vi "acqEngineHistoryStorage (U128).vi"(4 "ready for output":bool=TRUE, 7 "FIFO Out":refnum<k21>, 8 "PostTrigComplete":bool, 9 "AcqInProgress":bool, 10 "states":T1, 11 "Input Data":i16[](array[numeric])=[0, 0, 0, 0, 0, 0, 0, 0]) -> (0 "flushed":bool, 1 "valid":bool, 3 "Output Data":i16[](array[numeric]))   [LabVIEW 2011]
uses:
  <instrlib>/FlexRIO/Libraries/Acquisition Engine/FPGA/Interface/acqEngineStates v1.ctl
  <vilib>/rvi/DataTransferAndStorage/Container/Common/niFpgaContainerExecOnDevCompGetState.vi
  <vilib>/rvi/FIFO/Fifo_Resource/nirvififoEmulationSetSize.vi
  <vilib>/rvi/DataTransferAndStorage/Container/Common/niFpgaContainerGetUniqueNameForEmu.vi
  <vilib>/rvi/interface/RandomDataEmulation/nirviRandomDataFPGAFIFO.vi
  <vilib>/rvi/interface/RandomDataEmulation/niFpgaRandomDataHandleErrors.vi
  <vilib>/rvi/eio/common/nirviEmuReportErrorAndStop.vi
  <vilib>/rvi/FXPMathLib/basic elements/FxpDiscreteDelay/XNode/nifxpmath_DiscreteDelay.xnode
  <vilib>/rvi/DataTransferAndStorage/Container/XNode/niFpgaContainer.xnode
  <vilib>/rvi/FIFO/Fifo_Resource/niFpgaFifoEmulationRefIn.vi
  <instrlib>/FlexRIO/Libraries/Flexible Record Storage/Flexible Record Storage.lvlib
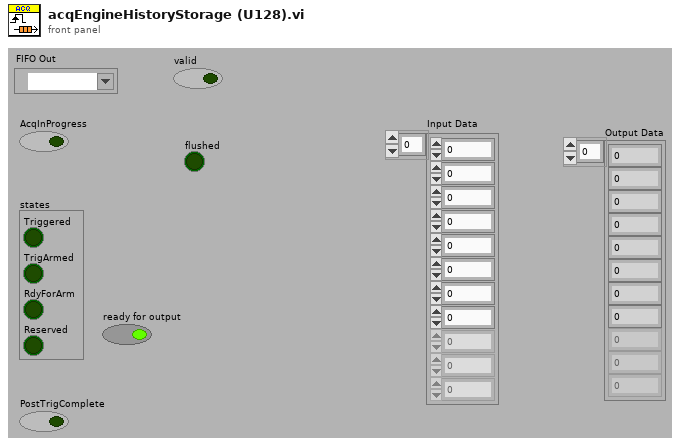
[diagram p1: front panel]
types:
  T1 = typedef "acqEngineStates v1.ctl" = cluster{"Triggered":bool, "TrigArmed":bool, "RdyForArm":bool, "Reserved":bool}
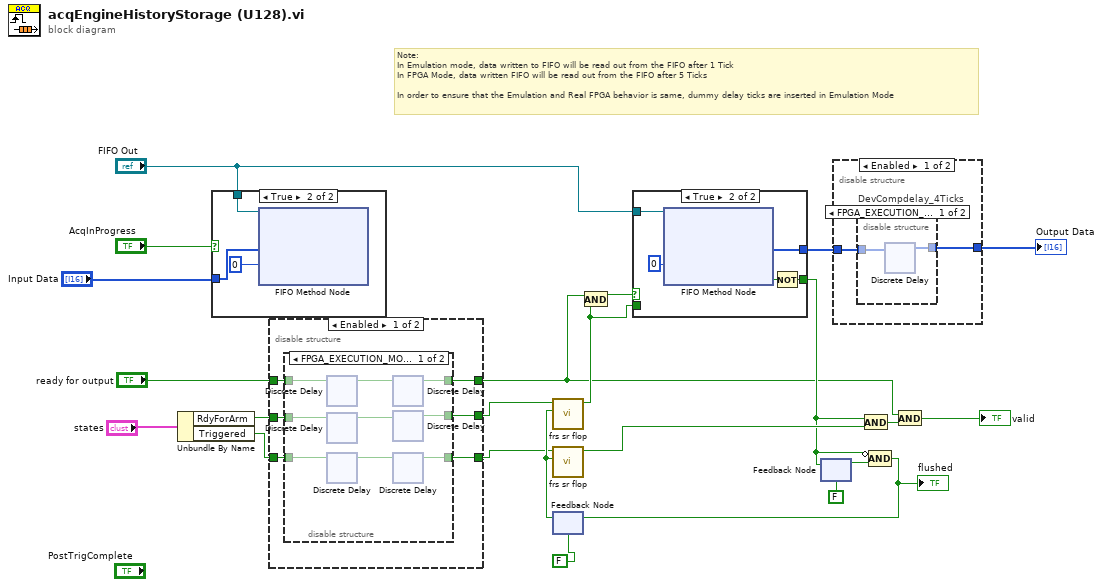
[diagram p0: block diagram]
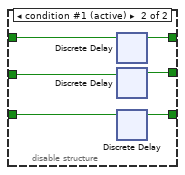
[diagram p2: hidden frame]
diagram:
  # "Note:\nIn Emulation mode, data written to FIFO will be read out from the FIFO after 1 Tick\nIn FPGA Mode, data written FIFO will be read out from the FIFO after 5 Ticks\n\nIn order to ensure that the Emulation and Real FPGA behavior is same, dummy delay ticks are inserted in Emulation Mode"
  n1 = Unbundle By Name("states") -> ("RdyForArm"=w19:bool, "Triggered"=w17:bool)
  n2 = case shown="True" "AcqInProgress" {
    tunnel: "FIFO Out" -> [_ w26]
    tunnel: "Input Data" -> [_ w25]
    frame False {
    }
    frame True {
      n3 = xnode ("FIFO Method Node")("Element"=w25, "Timeout"=0, "FIFO In"=w26) -> ()  [unwired: 2 out]
    }
  }
  n4 = disable-structure shown="Enabled" {
    disable-tunnel: w19 -> [w32 w49]
    disable-tunnel: w17 -> [w31 w48]
    disable-tunnel: "ready for output" -> [w30 w50]
    disable-tunnel: [w29 w49] -> w5
    disable-tunnel: [w28 w50] -> w4
    disable-tunnel: [w27 w48] -> w3
    frame Enabled {
      n5 = disable-structure shown="FPGA_EXECUTION_MODE==DEV_COMPUTER_SIM_IO, default" {
        disable-tunnel: w32 -> [w41 w47]
        disable-tunnel: w31 -> [w40 w46]
        disable-tunnel: w30 -> [w39 w45]
        disable-tunnel: [w38 w44] -> w29
        disable-tunnel: [w37 w43] -> w28
        disable-tunnel: [w36 w42] -> w27
        frame condition #0 {
          n6 = xnode "Discrete Delay"("D"=w39) -> ("Q"=w35:bool)
          n7 = xnode "Discrete Delay"("D"=w41) -> ("Q"=w34:bool)
          n8 = xnode "Discrete Delay"("D"=w40) -> ("Q"=w33:bool)
          n9 = xnode "Discrete Delay"("D"=w35) -> ("Q"=w37:bool)
          n10 = xnode "Discrete Delay"("D"=w34) -> ("Q"=w38:bool)
          n11 = xnode "Discrete Delay"("D"=w33) -> ("Q"=w36:bool)
        }
        frame condition #1 (active) {
          n12 = xnode "Discrete Delay"("D"=w45) -> ("Q"=w43:bool)
          n13 = xnode "Discrete Delay"("D"=w47) -> ("Q"=w44:bool)
          n14 = xnode "Discrete Delay"("D"=w46) -> ("Q"=w42:bool)
        }
      }
    }
    frame Disabled {
    }
  }
  n15 = feedback #1(FALSE) -> (w11:bool)
  n16 = call <instrlib>:"frs sr flop.vi"("r"=w11, "s"=w5) -> ("out"=w9:bool)  [unwired: 7 in]
  n17 = call <instrlib>:"frs sr flop.vi"("r"=w11, "s"=w3) -> ("out"=w16:bool)  [unwired: 7 in]
  n18 = And(x=w4, y=w9) -> (x .and. y?=w10:bool)
  n19 = case shown="True" w10 {
    tunnel: "FIFO Out" -> [_ w56]
    tunnel: [_ w55] -> w2
    tunnel: [w51 w54] -> w13
    tunnel: w9 -> [w51 _]
    frame False {
    }
    frame True {
      n20 = xnode ("FIFO Method Node")("Timeout"=0, "FIFO In"=w56) -> ("Element"=w55:i16[], "Timed Out?"=w53:bool)  [unwired: 1 out]
      n21 = Not(x=w53) -> (.not. x?=w54:bool)
    }
  }
  n22 = feedback #2(FALSE) -> (w15:bool)
  n23 = feedback-in #2(w13) -> ()
  n24 = disable-structure shown="Enabled" {
    disable-tunnel: w2 -> [w58 w62]
    disable-tunnel: [w57 w62] -> w1
    frame Enabled {
      n25 = disable-structure "DevCompdelay_4Ticks" shown="FPGA_EXECUTION_MODE==DEV_COMPUTER_SIM_IO, default" {
        disable-tunnel: w58 -> [w60 w61]
        disable-tunnel: [w59 w61] -> w57
        frame condition #0 {
          n26 = xnode "Discrete Delay"("D"=w60) -> ("Q"=w59:i16[])
        }
        frame condition #1 (active) {
        }
      }
    }
    frame Disabled {
    }
  }
  "Output Data" <- w1
  n27 = And(x=w13, y=w16) -> (x .and. y?=w18:bool)
  n28 = Compound Arithmetic op=AND(invert w13, w15) -> (w12:bool)
  "flushed" <- w12
  n29 = feedback-in #1(w12) -> ()
  n30 = And(x=w4, y=w18) -> (x .and. y?=→"valid":bool)
